vi "LED intensity control.vi"() -> ()   [LabVIEW 2023]
panel:
  in  "Write":bool
  in  "Exit":bool
  in  "Connect":bool
  in  "VISA resource name":refnum<visa-resource-name>
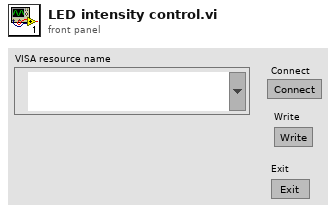
[diagram p1: front panel]
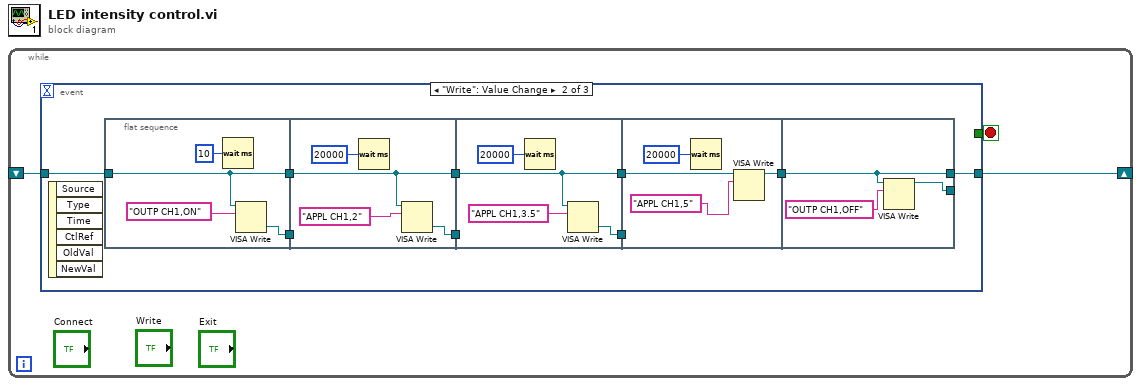
[diagram p0: block diagram]
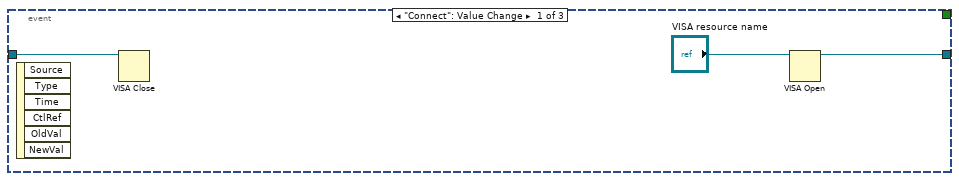
[diagram p2: hidden frame]
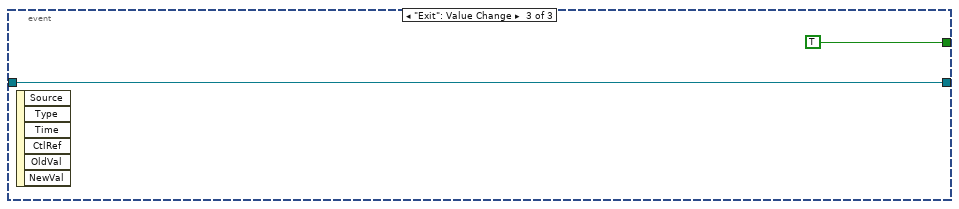
[diagram p3: hidden frame]
diagram:
  n1 = while {
    shift-right: [w1] -> _
    shift-left: _ -> [w3]
    stop <- w2 stop-if-true
    n2 = event shown="[1] \"Write\": Value Change" {
      selector: _ -> [_ _ _]
      dyn-events: _ -> [_ _ _]
      timeout: _ -> [_ _ _]
      tunnel: [w4 w15 w35] -> w1
      tunnel: w3 -> [w5 w14 w35]
      tunnel: [_ _ TRUE] -> w2
      event "Connect": Value Change {
        n3 = event-data() -> ()  [unwired: 1 in, 6 out]
        n4 = VISA Close(VISA resource name=w5) -> ()  [unwired: 1 in, 1 out]
        n5 = VISA Open(VISA resource name="VISA resource name") -> (VISA resource name=w4:refnum<visa-resource-name>)  [unwired: 4 in, 1 out]
      }
      event "Write": Value Change {
        n6 = event-data() -> ()  [unwired: 1 in, 6 out]
        n7 = flat-sequence {
          tunnel: w14 -> [w19]
          tunnel: [w19] -> w13
          tunnel: [w18] -> w12
          tunnel: [w22] -> w11
          tunnel: [w21] -> w10
          tunnel: w13 -> [w22]
          tunnel: w12 -> [_]
          tunnel: w11 -> [w27]
          tunnel: [w27] -> w9
          tunnel: w10 -> [_]
          tunnel: [w26] -> w8
          tunnel: w9 -> [w31]
          tunnel: w8 -> [_]
          tunnel: [w30] -> w7
          tunnel: [w34] -> w15
          tunnel: w7 -> [w34]
          tunnel: [w33] -> _
          frame #0 {
            n8 = Wait (ms)(milliseconds to wait=u32 10) -> ()  [unwired: 1 out]
            n9 = VISA Write(VISA resource name=w19, write buffer="OUTP CH1,ON") -> (VISA resource name out=w18:refnum<visa-resource-name>)  [unwired: 1 in, 2 out]
          }
          frame #1 {
            n10 = Wait (ms)(milliseconds to wait=u32 20000) -> ()  [unwired: 1 out]
            n11 = VISA Write(VISA resource name=w22, write buffer="APPL CH1,2") -> (VISA resource name out=w21:refnum<visa-resource-name>)  [unwired: 1 in, 2 out]
          }
          frame #2 {
            n12 = Wait (ms)(milliseconds to wait=u32 20000) -> ()  [unwired: 1 out]
            n13 = VISA Write(VISA resource name=w27, write buffer="APPL CH1,3.5") -> (VISA resource name out=w26:refnum<visa-resource-name>)  [unwired: 1 in, 2 out]
          }
          frame #3 {
            n14 = Wait (ms)(milliseconds to wait=u32 20000) -> ()  [unwired: 1 out]
            n15 = VISA Write(VISA resource name=w31, write buffer="APPL CH1,5") -> (VISA resource name out=w30:refnum<visa-resource-name>)  [unwired: 1 in, 2 out]
          }
          frame #4 {
            n16 = VISA Write(VISA resource name=w34, write buffer="OUTP CH1,OFF") -> (VISA resource name out=w33:refnum<visa-resource-name>)  [unwired: 1 in, 2 out]
          }
        }
      }
      event "Exit": Value Change {
        n17 = event-data() -> ()  [unwired: 1 in, 6 out]
      }
    }
  }
